vi "bh3_crc8.vi"(10 "polynomial(x8C)":u8=140 format="%02x", 11 "data payload":string) -> (2 "CRC-8 byte":u8 format="%02x", 3 "CRC-8 String":string)   [LabVIEW 2013]
panel:
  out "data_payload_bits":bool[](array[boolean])
  out "in2":bool[](array[boolean])
  out "input+zeros":bool[](array[boolean])
  out "divisor":bool[](array[boolean])
  out "result":bool[](array[boolean])
  out "CRC-8 bits":bool[](array[boolean])
  out "data_payload_bytes":u8[](array[numeric]) format="%02x"
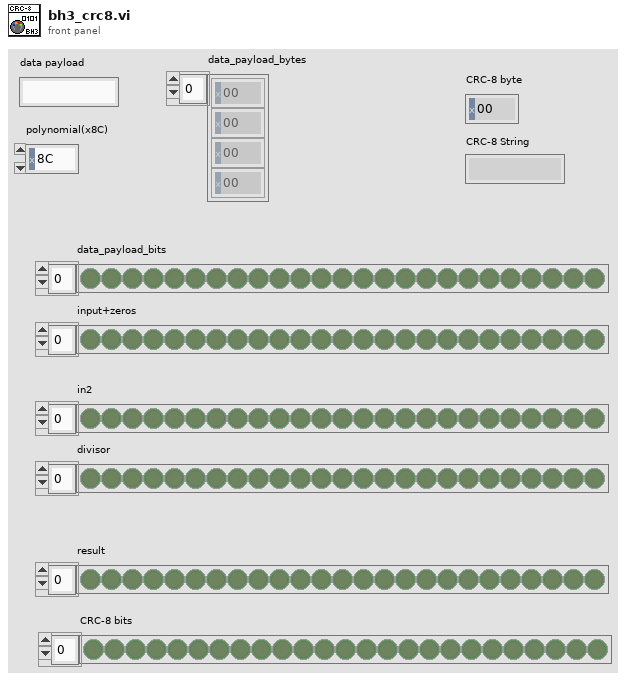
[diagram p1: front panel]
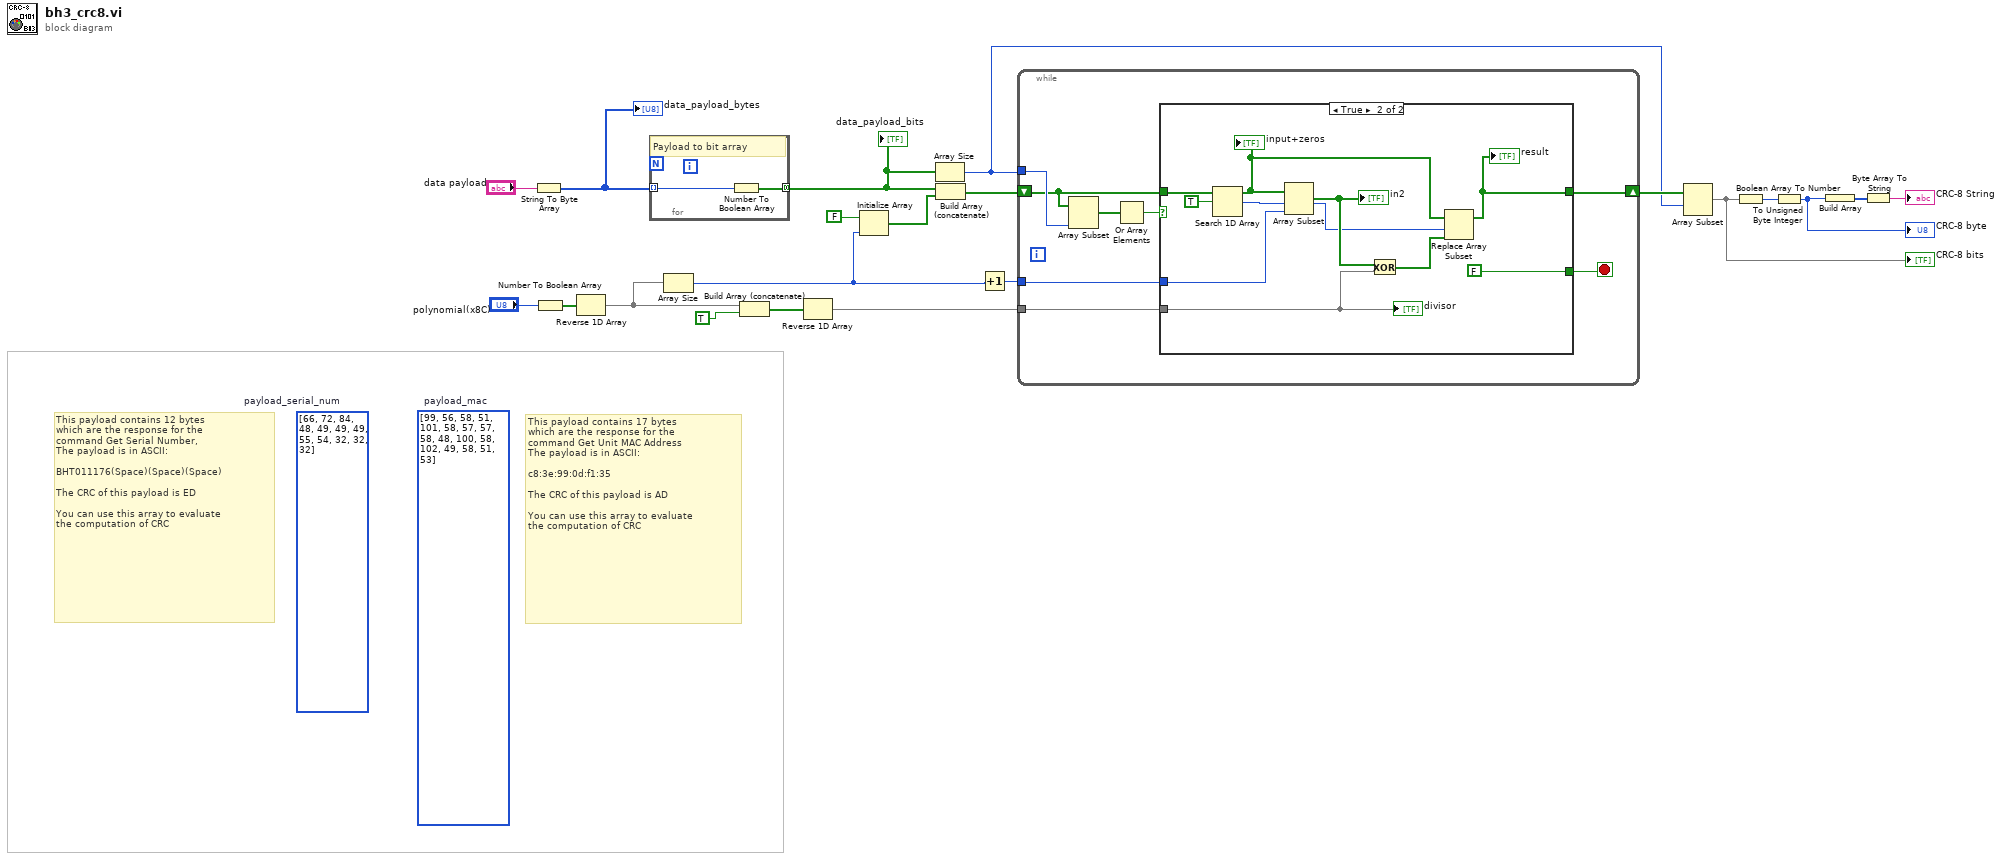
[diagram p0: block diagram]
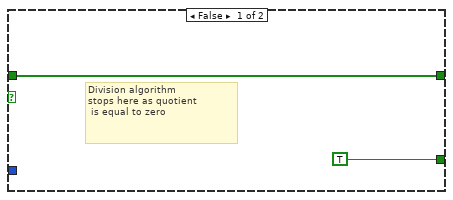
[diagram p2: hidden frame]
diagram:
  (unwired) u8[] [99, 56, 58, 51, 101, 58, 57, 57, 58, 48, 100, 58, 102, 49, 58, 51, 53]  # payload_mac
  (unwired) u8[] [66, 72, 84, 48, 49, 49, 49, 55, 54, 32, 32, 32]  # payload_serial_num
  # "This payload contains 17 bytes\nwhich are the response for the \ncommand Get Unit MAC Address \nThe payload is in ASCII:\n\nc8:3e:99:0d:f1:35\n\nThe CRC of this payload is AD\n\nYou can use this array to evaluate\nthe computation of CRC"
  # "This payload contains 12 bytes\nwhich are the response for the \ncommand Get Serial Number, \nThe payload is in ASCII:\n\nBHT011176(Space)(Space)(Space)\n\nThe CRC of this payload is ED\n\nYou can use this array to evaluate\nthe computation of CRC"
  n1 = String To Byte Array(string="data payload") -> (unsigned byte array=w1:u8[])
  "data_payload_bytes" <- w1
  n2 = Number To Boolean Array(number="polynomial(x8C)") -> (Boolean array=w11:bool[])
  n3 = Reverse 1D Array(array=w11) -> (reversed array=w10:bool[])
  n4 = for {
    tunnel: w1 -> [w23] mode=indexing
    tunnel: [w22] -> w7 mode=concatenating
    # "Payload to bit array"
    n5 = Number To Boolean Array(number=w23) -> (Boolean array=w22:bool[])
  }
  "data_payload_bits" <- w7
  n6 = Array Size(array=w10) -> (size(s)=w12:i32)
  n7 = Build Array (concatenate)(w10, TRUE) -> (w6:bool[])
  n8 = Reverse 1D Array(array=w6) -> (reversed array=w5:bool[])
  n9 = Initialize Array(FALSE, w12) -> (w18:bool[])
  n10 = Array Size(array=w7) -> (size(s)=w14:i32)
  n11 = Build Array (concatenate)(w7, w18) -> (w16:bool[])
  n12 = Increment(x=w12) -> (x+1=w13:i32)
  n13 = while {
    tunnel: w5 -> [w27]
    shift-right: [w28] -> w15
    shift-left: w16 -> [w26]
    tunnel: w13 -> [w31]
    tunnel: w14 -> [w29]
    stop <- w24 stop-if-true
    n14 = Array Subset(array=w26, length=w29) -> (w30:bool[])  [unwired: 1 in]
    n15 = Or Array Elements(Boolean array=w30) -> (logical OR=w25:bool)
    n16 = case shown="True" w25 {
      tunnel: w31 -> [_ w42]
      tunnel: [w33 w40] -> w28
      tunnel: w27 -> [_ w39]
      tunnel: w26 -> [w33 w35]
      tunnel: [TRUE FALSE] -> w24
      frame False {
        # "Division algorithm \nstops here as quotient\n is equal to zero"
      }
      frame True {
        n17 = Search 1D Array(1D array=w35, element=TRUE) -> (index of element=w36:i32)  [unwired: 1 in]
        n18 = Array Subset(array=w35, index=w36, length=w42) -> (w38:bool[])
        "in2" <- w38
        n19 = Exclusive Or(1:w39, 2:w38) -> (0:w41:bool[])
        n20 = Replace Array Subset(array=w35, new element=w41, index=w36) -> (w40:bool[])
        "result" <- w40
        "divisor" <- w39
        "input+zeros" <- w35
      }
    }
  }
  n21 = Array Subset(array=w15, index=w14) -> (w8:bool[])  [unwired: 1 in]
  "CRC-8 bits" <- w8
  n22 = Boolean Array To Number(Boolean array=w8) -> (number=w4:u32)
  n23 = To Unsigned Byte Integer(number=w4) -> (unsigned 8bit integer=w3:u8)
  "CRC-8 byte" <- w3
  n24 = Build Array(w3) -> (w2:u8[])
  n25 = Byte Array To String(unsigned byte array=w2) -> (string=→"CRC-8 String":string)
